vi "DiffDrivePoseEst_New.vi"(4 "RightDistance_M":dbl=0.02, 5 "gyroAngle":T4={"VALUE"=0.0, "COS"=1.0, "SIN"=0.0} {"SIN" format="%13.4f"; "COS" format="%13.4f"; "VALUE" format="%13.4f"}, 6 "LeftDistance_M":dbl=0.02, 7 "InitialPose":T2={"TRANSLATION"={"X"=0.0, "Y"=0.0}, "ROTATION"={"VALUE"=0.0, "COS"=1.0, "SIN"=0.0}} {"ROTATION"."SIN" format="%13.4f"; "ROTATION"."COS" format="%13.4f"; "ROTATION"."VALUE" format="%13.4f"; "TRANSLATION"."Y" format="%14.3f"; "TRANSLATION"."X" format="%14.3f"}, 8 "dt_Seconds":dbl=0.02, 9 "VisionMeasurementStdDevs":T1, 10 "LocalMeasurementStdDevs":T1, 11 "StateStdDevs":T1) -> (0 "Error":errorcluster, 3 "DiffDrivePoseEstimate":T5={"M_VisionContR"=[], "m_nominal_dT"=0.0, "m_PrevTime_Sec"=0.0, "m_GyroOffset"={"VALUE"=0.0, "COS"=1.0, "SIN"=0.0}, "m_PrevAngle"={"VALUE"=0.0, "COS"=1.0, "SIN"=0.0}, "StartLeftEnc_M"=0.0, "StartRightEnc_M"=0.0, "m_Observer"={"m_P"=[], "m_xHat"=[], "States"=0, "Outputs"=0, "m_ContR"=[], "m_ContQ"=[], "m_SigmasF"=[], "m_dT_Sec"=0.0, "MERWE_SCALED_SIGMA_PTS"={"m_Wm"=[], "States"=0, "Alpha"=0.0, "m_Wc"=[], "Kappa"=0}, "meanFuncX"=refnum, "meanFuncY"=refnum, "residualFuncX"=refnum, "residualFuncY"=refnum, "addFuncX"=refnum, "addFuncXExtra"=variant, "residualFuncYExtra"=variant, "residualFuncXExtra"=variant, "MeanFuncYExtra"=variant, "MeanFuncXExtra"=variant, "Inputs"=0}, "Pose_Buffer"={"TimeStamps"=[], "Pose"=[], "Min_TimeStamp"=0.0, "Max_TimeStamp"=0.0, "ItemCount"=0, "MaxBufferTime"=0.0}} {"Pose_Buffer"."Pose"."ROTATION"."SIN" format="%13.4f"; "Pose_Buffer"."Pose"."ROTATION"."COS" format="%13.4f"; "Pose_Buffer"."Pose"."ROTATION"."VALUE" format="%13.4f"; "Pose_Buffer"."Pose"."TRANSLATION"."Y" format="%14.3f"; "Pose_Buffer"."Pose"."TRANSLATION"."X" format="%14.3f"; "m_PrevAngle"."SIN" format="%13.4f"; "m_PrevAngle"."COS" format="%13.4f"; "m_PrevAngle"."VALUE" format="%13.4f"; "m_GyroOffset"."SIN" format="%13.4f"; "m_GyroOffset"."COS" format="%13.4f"; "m_GyroOffset"."VALUE" format="%13.4f"})   [LabVIEW 2019, in "Trajectory_Library.lvlib"]
doc: "This set of functions is deprecated. Suggest using the new Diff Drive Pose Est 2 instead.\n\nThis set of subVI wraps an UnscentedKalmanFilter to fuse latency-compensated vision measurements with differential drive encoder measurements. It will correct for noisy vision measurements and encoder drift. It is intended to be an easy drop-in for {@link edu.wpi.first.math.kinematics.DifferentialDriveOdometry}; in fact, if you never call DifferentialDrivePoseEstimator_addVisionMeasurement and only call DifferentialDrivePoseEstimator_update then this will behave exactly the same as DifferentialDriveOdometry.\n \nDifferentialDrivePoseEstimator_update}should be called every robot loop (if your robot loops are faster than the default then you should change the DifferentialDrivePoseEstimator_DifferentialDrivePoseEstimator(Rotation2d, Pose2d, Matrix, Matrix,\nMatrix, double) nominal delta time.) DifferentialDrivePoseEstimator_addVisionMeasurement can be called as infrequently as you want; if you never call it then this class will behave exactly like regular encoder odometry.\n\nTo promote stability of the pose estimate and make it robust to bad vision data, we recommend only adding vision measurements that are already within one meter or so of the current pose estimate.\n\nOur state-space system is:\n\n x = [[x, y, theta, dist_l, dist_r]]? in the field coordinate system (dist_* are wheel distances.)\n \n u = [[vx, vy, omega]]? (robot-relative velocities) -- NB: using velocities make things considerably easier, because it means that teams don't have to worry about getting an accurate model. Basically, we suspect that it's easier for teams to get good encoder data than it is for them to perform system identification well enough to get a good model.\n \n y = [[x, y, theta]]? from vision, or <strong>y = [[dist_l, dist_r, theta]] from encoders and gyro.\n \nConstructs a DifferentialDrivePoseEstimator.\n\nInputs\n - gyroAngle -- The current gyro angle. (radians)\n - initialPoseMeters -- The starting pose estimate.\n - stateStdDevs -- Standard deviations of model states. Increase these numbers to trust your\n model's state estimates less. This matrix is in the form [x, y, theta, dist_l, dist_r]?,\n with units in meters and radians.\n - localMeasurementStdDevs -- Standard deviations of the encoder and gyro measurements.\n Increase these numbers to trust sensor readings from encoders and gyros less. This matrix\n is in the form [dist_l, dist_r, theta]?, with units in meters and radians.\n - visionMeasurementStdDevs -- Standard deviations of the vision measurements. Increase these\n numbers to trust global measurements from vision less. This matrix is in the form [x, y,\n theta]?, with units in meters and radians.\n - nominalDtSeconds -- The time in seconds between each robot loop. (seconds)\n - leftDistance_M -- The initial left wheel distance measurement (meters)\n - rightDistance_M -- The initial right wheel distance measurement (meters)\n\nOutputs:\n - DiffDrivePoseEst -- Data cluster for this instance of this system.\n - Error -- A value of TRUE indicates an error occured creating the system."
uses:
  Trajectory_Library.lvlib
  TypeDef/DIFF_DRIVE_POSE_EST.ctl
  <vilib>/Analysis/Matrix/Datatypes/RealMatrix.ctl
  TypeDef/ROTATION2D.ctl
  TypeDef/UNSCENTED_KALMAN_FILTER.ctl
  TypeDef/MERWE_SCALED_SIGMA_PTS.ctl
  TypeDef/CALLBACK_FUNC_TYPE.ctl
  TypeDef/TIME_INTERPOLATABLE_POSE2D.ctl
  TypeDef/POSE2D.ctl
  TypeDef/TRANSLATION2D.ctl
  MatBuilder_Create.vi
  Rotation2d_UnaryMinus.vi
  Rotation2d_RotateBy.vi
  Rotation2d_CreateAngle.vi
  Rotation2d_CreateXY.vi
  Util_CalcDist.vi
  <vilib>/Analysis/Matrix/NI_Matrix.lvlib
panel:
  # "<5,1>"
  # "<3, 1>"
  # "<3, 1>"
  # "<3, 3>"
  # "State Estimate <Statess,1>"
  # "<States, States>"
  # "<States, ?>"
  # "<Statess,  States>"
  # "<Outputs, Outputs>"
  # "<?, 1>"
  # "<?, 1>"
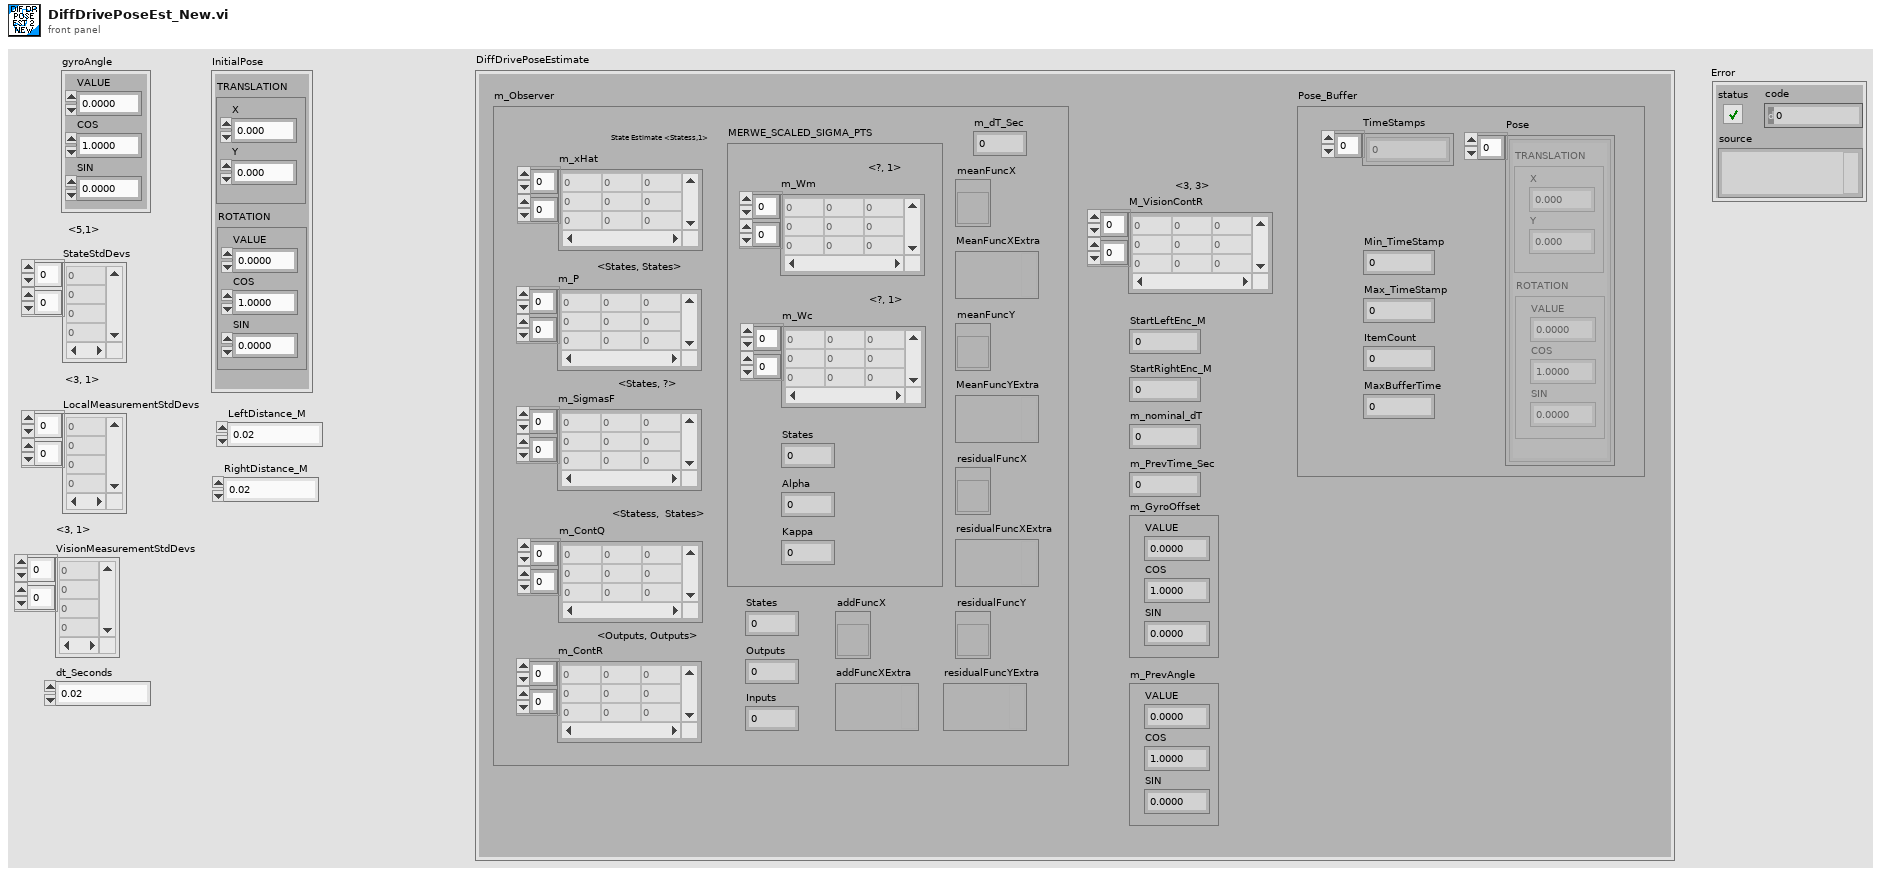
[diagram p1: front panel]
types:
  T1 = typedef "NI_Matrix.lvlib/RealMatrix.ctl" = dbl[][]
  T2 = typedef "Trajectory_Library.lvlib/POSE2D.ctl" = cluster{"TRANSLATION":T3, "ROTATION":T4}
  T3 = typedef "Trajectory_Library.lvlib/TRANSLATION2D.ctl" = cluster{"X":dbl, "Y":dbl}
  T4 = typedef "Trajectory_Library.lvlib/ROTATION2D.ctl" = cluster{"VALUE":dbl, "COS":dbl, "SIN":dbl}
  T5 = typedef "Trajectory_Library.lvlib/DIFF_DRIVE_POSE_EST.ctl" = cluster{"M_VisionContR":T1, "m_nominal_dT":dbl, "m_PrevTime_Sec":dbl, "m_GyroOffset":T4, "m_PrevAngle":T4, "StartLeftEnc_M":dbl, "StartRightEnc_M":dbl, "m_Observer":T6, "Pose_Buffer":T9}
  T6 = typedef "Trajectory_Library.lvlib/UNSCENTED_KALMAN_FILTER.ctl" = cluster{"m_P":T1, "m_xHat":T1, "States":i32, "Outputs":i32, "m_ContR":T1, "m_ContQ":T1, "m_SigmasF":T1, "m_dT_Sec":dbl, "MERWE_SCALED_SIGMA_PTS":T7, "meanFuncX":T8, "meanFuncY":T8, "residualFuncX":T8, "residualFuncY":T8, "addFuncX":T8, "addFuncXExtra":variant, "residualFuncYExtra":variant, "residualFuncXExtra":variant, "MeanFuncYExtra":variant, "MeanFuncXExtra":variant, "Inputs":i32}
  T7 = typedef "Trajectory_Library.lvlib/MERWE_SCALED_SIGMA_PTS.ctl" = cluster{"m_Wm":T1, "States":i32, "Alpha":dbl, "m_Wc":T1, "Kappa":i32}
  T8 = typedef "Trajectory_Library.lvlib/CALLBACK_FUNC_TYPE.ctl" = refnum<vi>
  T9 = typedef "Trajectory_Library.lvlib/TIME_INTERPOLATABLE_POSE2D.ctl" = cluster{"TimeStamps":dbl[], "Pose":T2[], "Min_TimeStamp":dbl, "Max_TimeStamp":dbl, "ItemCount":i32, "MaxBufferTime":dbl}
  T10 = typedef "Trajectory_Library.lvlib/UNSCENTED_KALMAN_NEW_FUNC_GROUP.ctl" = cluster{"meanFuncX":T8, "meanFuncY":T8, "residualFuncX":T8, "residualFuncY":T8, "addFuncX":T8, "MeanFuncXExtra":variant, "MeanFuncYExtra":variant, "residualFuncXExtra":variant, "residualFuncYExtra":variant, "addFuncXExtra":variant}
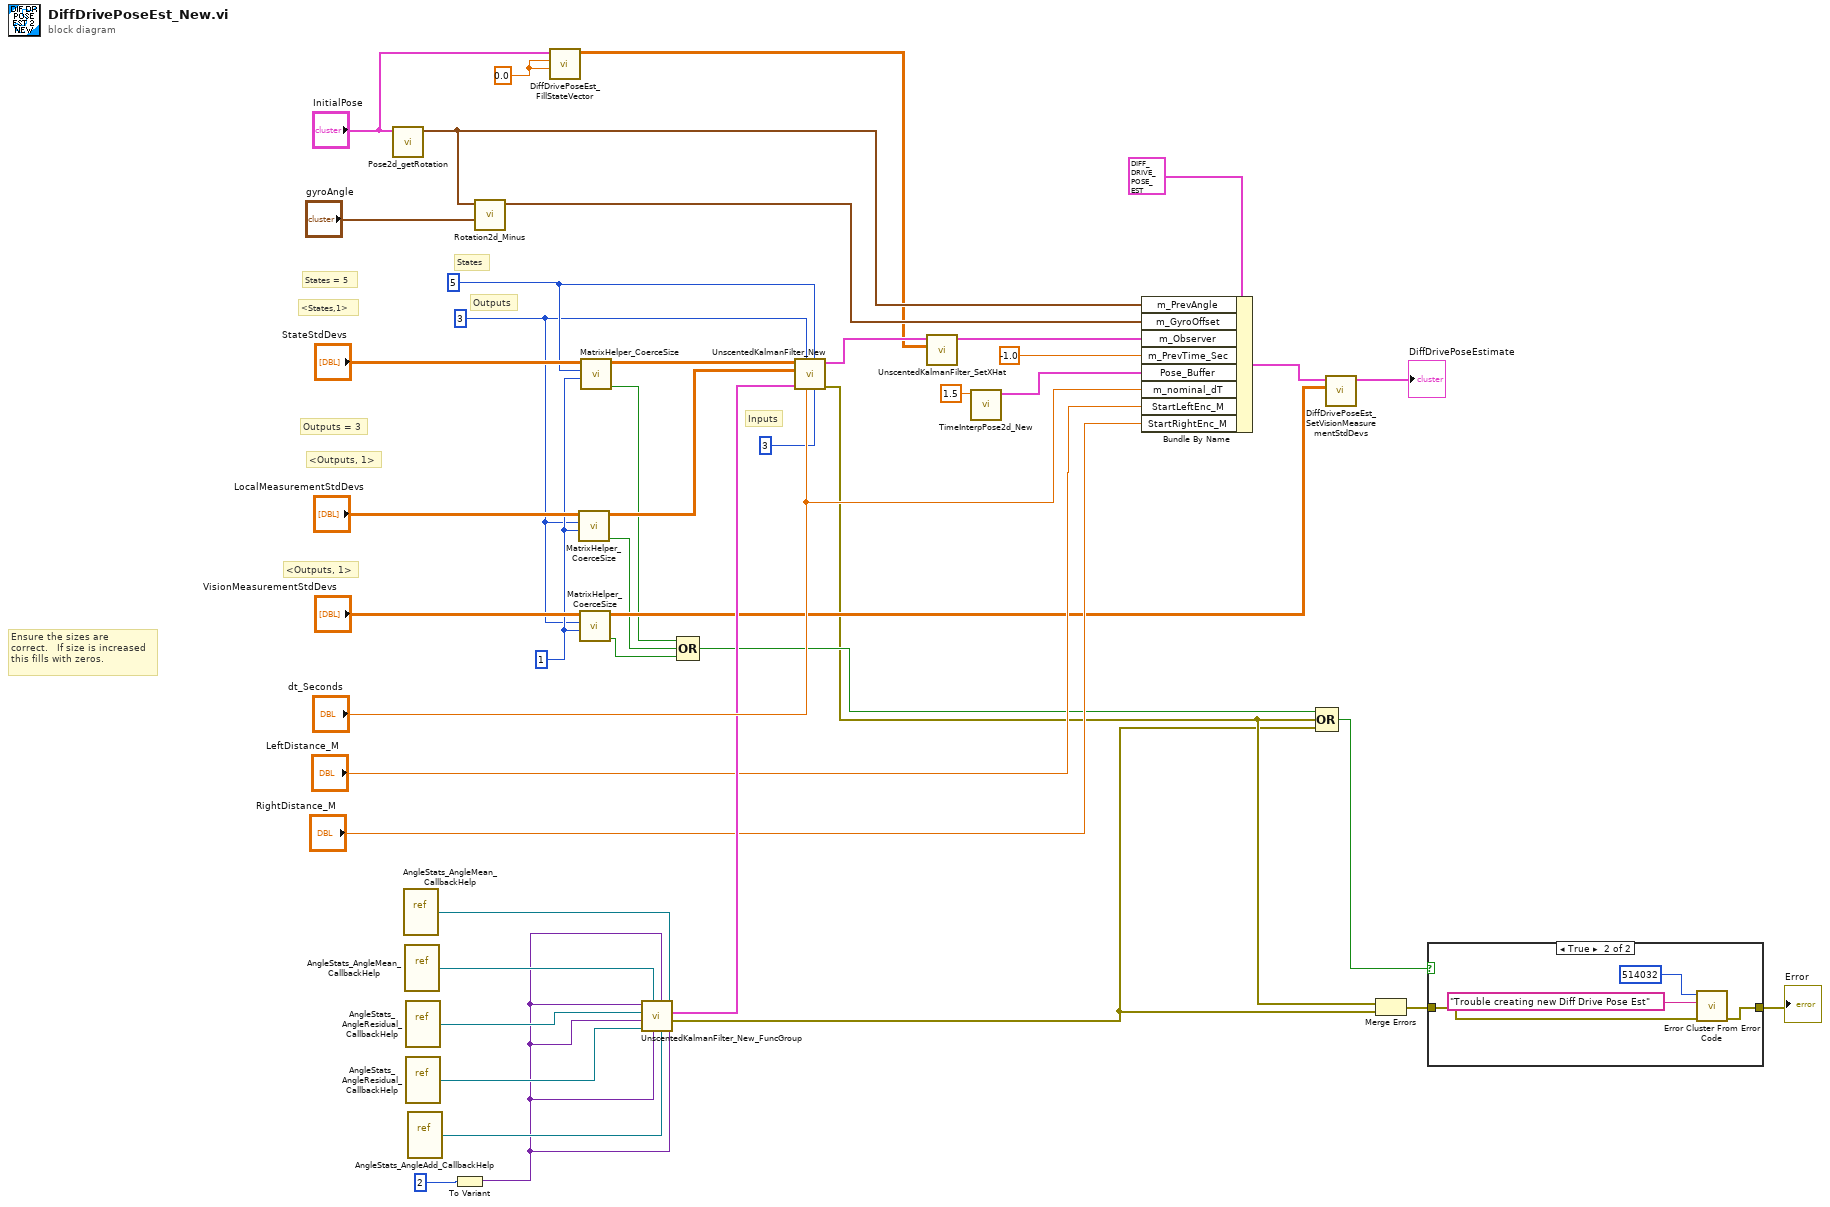
[diagram p0: block diagram]
diagram:
  w14 = 1 ("y")
  w36 = 0.0 ("LeftDist")
  w12 = 3 ("Outputs")
  w13 = 5 ("States")
  # "Inputs"
  # "<Outputs, 1>"
  # "Outputs = 3"
  # "States = 5"
  # "Outputs"
  # "States"
  # "<Outputs, 1>"
  # "<States,1>"
  # "Ensure the sizes are\ncorrect.   If size is increased \nthis fills with zeros."
  n1 = call "Pose2d_getRotation.vi"("in POSE"="InitialPose") -> ("out ROTATION"=w40:T4)  [unwired: 10 in]
  n2 = vi-ref "AngleStats_AngleMean_CallbackHelp.vi"() -> (w30:refnum<vi>)
  n3 = vi-ref "AngleStats_AngleMean_CallbackHelp.vi"() -> (w29:refnum<vi>)
  n4 = vi-ref "AngleStats_AngleResidual_CallbackHelp.vi"() -> (w28:refnum<vi>)
  n5 = vi-ref "AngleStats_AngleResidual_CallbackHelp.vi"() -> (w27:refnum<vi>)
  n6 = vi-ref "AngleStats_AngleAdd_CallbackHelp.vi"() -> (w25:refnum<vi>)
  n7 = To Variant(anything=2) -> (Variant=w24:variant)
  n8 = call "Rotation2d_Minus.vi"("other ROTATION"="gyroAngle", "in ROTATION"=w40) -> ("out ROTATION"=w41:T4)  [unwired: 9 in]
  n9 = call "DiffDrivePoseEst_FillStateVector.vi"("RightDist"=w36, "LeftDist"=w36, "InitialPose"="InitialPose") -> ("output matrix"=w35:T1)  [unwired: 8 in]
  n10 = call "MatrixHelper_CoerceSize.vi"("Columns"=w14, "Rows"=w12, "input matrix"="LocalMeasurementStdDevs") -> ("Coerced"=w9:bool, "output matrix"=w19:T1)  [unwired: 7 in]
  n11 = call "MatrixHelper_CoerceSize.vi"("Columns"=w14, "Rows"=w12, "input matrix"="VisionMeasurementStdDevs") -> ("Coerced"=w8:bool, "output matrix"=w15:T1)  [unwired: 7 in]
  n12 = call "MatrixHelper_CoerceSize.vi"("Columns"=w14, "Rows"=w13, "input matrix"="StateStdDevs") -> ("Coerced"=w10:bool, "output matrix"=w17:T1)  [unwired: 7 in]
  n13 = call "UnscentedKalmanFilter_New_FuncGroup.vi"("addFuncXExtra"=w24, "MeanFuncX"=w30, "AddFuncX"=w25, "MeanFuncXExtra"=w24, "residualFuncYExtra"=w24, "MeanFuncY"=w29, "ResidualFuncY"=w27, "residualFuncXExtra"=w24, "ResidualFuncX"=w28, "MeanFuncYExtra"=w24) -> ("Error"=w4:errorcluster, "UNSCENTED_KALMAN_NEW_FUNC_GROUP"=w31:T10)
  n14 = Compound Arithmetic op=OR(w10, w9, w8) -> (w11:bool)
  n15 = call "UnscentedKalmanFilter_New.vi"("Inputs"=3, "States"=w13, "dt_Seconds"="dt_Seconds", "Outputs"=w12, "UNSCENTED_KALMAN_NEW_FUNC_GROUP"=w31, "MeasurementStdDevs"=w19, "StateStdDevs"=w17) -> ("Error"=w5:errorcluster, "UnscentedKalmanFiilter"=w38:T6)  [unwired: 3 in]
  n16 = call "UnscentedKalmanFilter_SetXHat.vi"("xHat"=w35, "in UnscentedKalmanFiilter"=w38) -> ("out UnscentedKalmanFiilter"=w39:T6)  [unwired: 8 in, 1 out]
  n17 = call "TimeInterpPose2d_New.vi"("MaxTime"=1.5) -> ("TimeInterpPose"=w1:T9)  [unwired: 10 in]
  n18 = Bundle By Name(cluster=T5 {"M_VisionContR"=[], "m_nominal_dT"=0.0, "m_PrevTime_Sec"=0.0, "m_GyroOffset"={"VALUE"=0.0, "COS"=1.0, "SIN"=0.0}, "m_PrevAngle"={"VALUE"=0.0, "COS"=1.0, "SIN"=0.0}, "StartLeftEnc_M"=0.0, "StartRightEnc_M"=0.0, "m_Observer"={"m_P"=[], "m_xHat"=[], "States"=0, "Outputs"=0, "m_ContR"=[], "m_ContQ"=[], "m_SigmasF"=[], "m_dT_Sec"=0.0, "MERWE_SCALED_SIGMA_PTS"={"m_Wm"=[], "States"=0, "Alpha"=0.0, "m_Wc"=[], "Kappa"=0}, "meanFuncX"=refnum, "meanFuncY"=refnum, "residualFuncX"=refnum, "residualFuncY"=refnum, "addFuncX"=refnum, "addFuncXExtra"=variant, "residualFuncYExtra"=variant, "residualFuncXExtra"=variant, "MeanFuncYExtra"=variant, "MeanFuncXExtra"=variant, "Inputs"=0}, "Pose_Buffer"={"TimeStamps"=[], "Pose"=[], "Min_TimeStamp"=0.0, "Max_TimeStamp"=0.0, "ItemCount"=0, "MaxBufferTime"=0.0}} ("DIFF_DRIVE_POSE_EST"), "m_PrevAngle"=w40, "m_GyroOffset"=w41, "m_Observer"=w39, "m_PrevTime_Sec"=-1.0, "Pose_Buffer"=w1, "m_nominal_dT"="dt_Seconds", "StartLeftEnc_M"="LeftDistance_M", "StartRightEnc_M"="RightDistance_M") -> (w34:T5)
  n19 = Compound Arithmetic op=OR(w11, w5, w4) -> (w7:bool)
  n20 = call "DiffDrivePoseEst_SetVisionMeasurementStdDevs.vi"("VisionMeasurementStdDevs"=w15, "in DiffDrivePoseEstimate"=w34) -> ("Out DiffDrivePoseEstimate"=→"DiffDrivePoseEstimate":T5)  [unwired: 8 in, 1 out]
  n21 = Merge Errors(w5, w4) -> (w6:errorcluster)
  n22 = case shown="True" w7 {
    tunnel: w6 -> [w45 w48]
    tunnel: [w45 w49] -> w3
    frame False {
    }
    frame True {
      n23 = call <vilib>:"Error Cluster From Error Code.vi"("error in (no error)"=w48, "error message (\"\")"="Trouble creating new Diff Drive Pose Est" ("error message (\"\")"), "error code (0)"=514032) -> ("error out"=w49:errorcluster)  [unwired: 6 in]
    }
  }
  "Error" <- w3
